vi "ReversedEngineering CreateStateTransationEdges.vi"(1 "GraphRefToAddNodesTo":refnum<class "Graph.lvclass">, 2 "StateDiagramReverseOptions":T1={"Clear All Current States"=TRUE, "UseMenuItem"=TRUE, "InsertArrayQueuedElementsVI"="", "Add Actions"=FALSE, "StateDiagramSerachActions"={"Action"=enum."NotTheseVIs", "VINames"=[], "LimitActions(VIs)"=10}, "AddCaseCommentsAsActions"=FALSE, "IgnoreStatesNotUsed"=FALSE, "CommentsSerachActions"={"MinimumTextLength"=0, "OnlyTopLeftComment"=FALSE, "CommentPrefix"=""}, "TransitionMode"=enum."Add to current transtion text", "ActionMode"=enum."Add to current action text"}, 3 "States":T5[](array[typedef]), 5 "error in (no error)":errorcluster, 7 "graphics":refnum<class "Graphics.lvclass">, 9 "grid":refnum<class "Grid.lvclass">) -> (19 "error out":errorcluster)   [LabVIEW 2014]
uses:
  <resource>/Framework/Providers/Open_GDS/UML/ReversedEngineering/ReversedEngineering StateMachineStateInfo.ctl
  <resource>/Framework/Providers/Open_GDS/UML/Graph_class/Graph.lvclass
  <resource>/Framework/Providers/Open_GDS/UML/Graphics_class/Graphics.lvclass
  <resource>/Framework/Providers/Open_GDS/UML/Grid_class/Grid.lvclass
  <resource>/Framework/Providers/Open_GDS/UML/ReversedEngineering/private/ReversedEngineering StateDiagramReverseOptions.ctl
  <resource>/Framework/Providers/Open_GDS/UML/ReversedEngineering/private/ReversedEngineering StateDiagramSerachActions.ctl
  <resource>/Framework/Providers/Open_GDS/UML/ReversedEngineering/ReversedEngineering StateAnalyseVIAction.ctl
  <resource>/Framework/Providers/Open_GDS/UML/ReversedEngineering/private/ReversedEngineering StateDiagramCommentSearchType.ctl
  <resource>/Framework/Providers/Open_GDS/UML/AbstractEdge_class/AbstractEdge.lvclass
  <resource>/Framework/Providers/Open_GDS/UML/StateNode_class/StateNode.lvclass
  <resource>/Framework/Providers/Open_GDS/UML/StateTransitionEdge_class/StateTransitionEdge.lvclass
  <resource>/Framework/Providers/Open_GDS/UML/MultiLineString_class/MultiLineString.lvclass
  <resource>/Framework/Providers/Open_GDS/UML/AbstractNode_class/AbstractNode.lvclass
  <resource>/Framework/Providers/Open_GDS/UML/StateReverse_class/StateReverse.lvclass
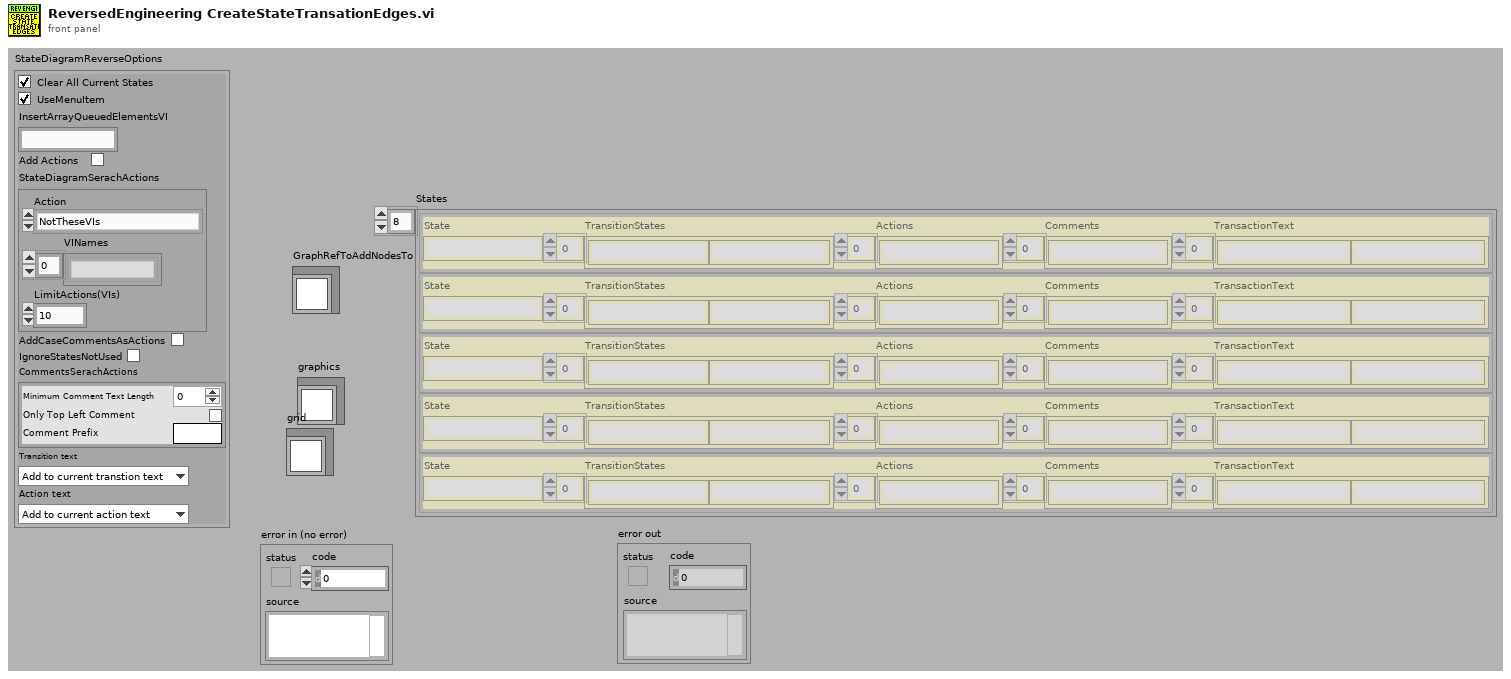
[diagram p1: front panel]
types:
  T1 = typedef "ReversedEngineering StateDiagramReverseOptions.ctl" = cluster{"Clear All Current States":bool, "UseMenuItem":bool, "InsertArrayQueuedElementsVI":string, "Add Actions":bool, "StateDiagramSerachActions":T2, "AddCaseCommentsAsActions":bool, "IgnoreStatesNotUsed":bool, "CommentsSerachActions":T4, "TransitionMode":enum16{"Add to current transtion text", "Replace transition text"}, "ActionMode":enum16{"Add to current action text", "Replace action text"}}
  T2 = typedef "ReversedEngineering StateDiagramSerachActions.ctl" = cluster{"Action":T3, "VINames":string[], "LimitActions(VIs)":i32}
  T3 = typedef "ReversedEngineering StateAnalyseVIAction.ctl" = enum16{"OnlyTheseVIs", "NotTheseVIs"}
  T4 = typedef "ReversedEngineering StateDiagramCommentSearchType.ctl" = cluster{"MinimumTextLength":i32, "OnlyTopLeftComment":bool, "CommentPrefix":string}
  T5 = typedef "ReversedEngineering StateMachineStateInfo.ctl" = cluster{"State":string, "TransitionStates":string[], "Actions":string[], "Comments":string[], "TransactionText":string[]}
  T6 = enum16{"Add to current transtion text", "Replace transition text"}
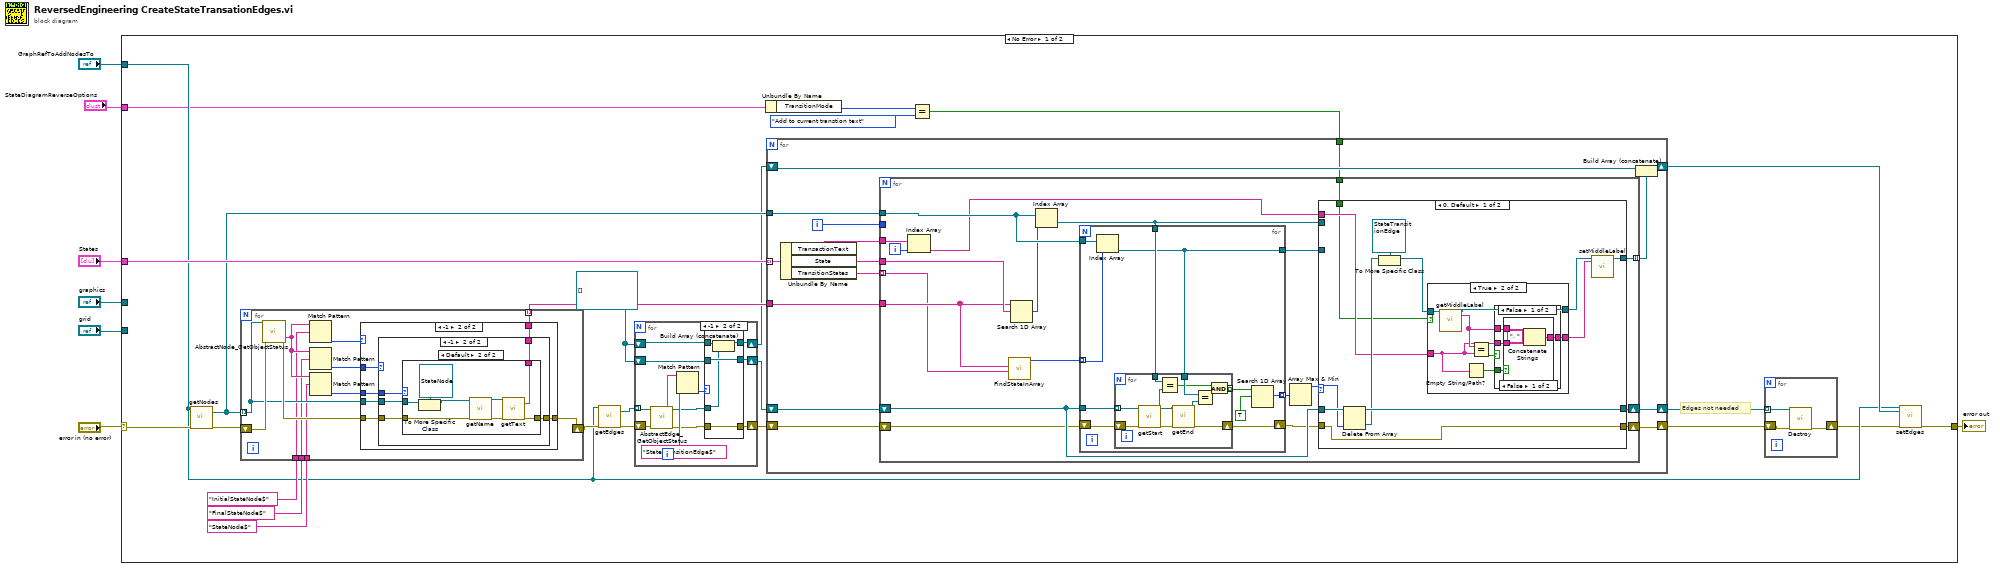
[diagram p0: block diagram]
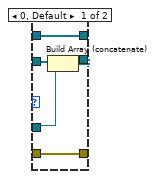
[diagram p2: hidden frame]
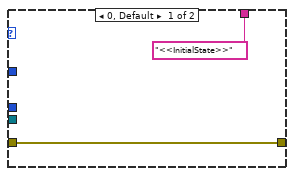
[diagram p3: hidden frame]
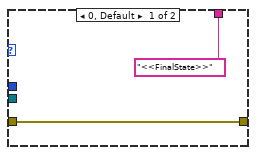
[diagram p4: hidden frame]
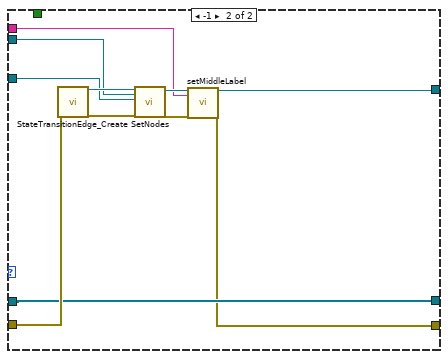
[diagram p9: hidden frame]
diagram:
  n1 = case shown="No Error" "error in (no error)" {
    selector: "error in (no error)" -> [w32 w193]
    tunnel: [w31 w193] -> w6
    tunnel: "States" -> [w30 _]
    tunnel: "GraphRefToAddNodesTo" -> [w21 _]
    tunnel: "graphics" -> [_ _]
    tunnel: "grid" -> [_ _]
    tunnel: "StateDiagramReverseOptions" -> [w11 _]
    frame No Error {
      w13 = refnum<class "AbstractEdge.lvclass">[] []
      # "Edges not needed"
      n2 = call-dynamic "getNodes.vi"("reference"=w21, "error in (no error)"=w32) -> ("nodes"=w29:refnum<class "AbstractNode.lvclass">[], "error out"=w24:errorcluster)  [unwired: 15 in, 1 out]
      n3 = for {
        shift-right: [w66] -> w22
        shift-left: w24 -> [w67]
        tunnel: w29 -> [w64] mode=indexing
        tunnel: [w65] -> w28 mode=indexing
        tunnel: "StateNode$" -> [w63]
        tunnel: "FinalStateNode$" -> [w61]
        tunnel: "InitialStateNode$" -> [w60]
        n4 = call <resource>:"AbstractNode_GetObjectStatus.vi"("reference in"=w64, "error in (no error)"=w67) -> ("Class name"=w62:string, "error out"=w69:errorcluster)  [unwired: 16 out]
        n5 = Match Pattern(string=w62, regular expression=w60) -> (offset past match=w59:i32)  [unwired: 4 out]
        n6 = Match Pattern(string=w62, regular expression=w61) -> (offset past match=w58:i32)  [unwired: 4 out]
        n7 = Match Pattern(string=w62, regular expression=w63) -> (offset past match=w68:i32)  [unwired: 4 out]
        n8 = case shown="-1" w59 {
          tunnel: w69 -> [w70 w77]
          tunnel: w68 -> [_ w76]
          tunnel: [w70 w75] -> w66
          tunnel: ["<<InitialState>>" ("text") w74] -> w65
          tunnel: w64 -> [_ w73]
          tunnel: w58 -> [_ w72]
          frame 0, Default {
          }
          frame -1 {
            n9 = case shown="-1" w72 {
              tunnel: w77 -> [w78 w84]
              tunnel: w76 -> [_ w83]
              tunnel: [w78 w82] -> w75
              tunnel: ["<<FinalState>>" ("text") w81] -> w74
              tunnel: w73 -> [_ w80]
              frame 0, Default {
              }
              frame -1 {
                n10 = case shown="Default" w83 {
                  tunnel: w80 -> [_ w88]
                  tunnel: w84 -> [w85 w93]
                  tunnel: [w85 w90] -> w82
                  tunnel: [_ w89] -> w81
                  frame -1 {
                  }
                  frame Default {
                    n11 = To More Specific Class(target class=refnum<class "StateNode.lvclass"> refnum ("reference"), reference=w88) -> (specific class reference=w86:refnum<class "StateNode.lvclass">)  [unwired: 1 in, 1 out]
                    n12 = call-dynamic "getName.vi"("reference"=w86, "error in (no error)"=w93) -> ("name"=w92:refnum<class "MultiLineString.lvclass">, "error out"=w91:errorcluster)  [unwired: 15 in, 1 out]
                    n13 = call-dynamic "getText.vi"("reference"=w92, "error in (no error)"=w91) -> ("text"=w89:string, "error out"=w90:errorcluster)  [unwired: 15 in, 1 out]
                  }
                }
              }
            }
          }
        }
      }
      n14 = call-dynamic "getEdges.vi"("reference"=w21, "error in (no error)"=w22) -> ("edges"=w16:refnum<class "AbstractEdge.lvclass">[], "error out"=w17:errorcluster)  [unwired: 15 in, 1 out]
      n15 = for {
        tunnel: w16 -> [w44] mode=indexing
        shift-right: [w39] -> w14
        shift-left: w17 -> [w43]
        shift-right: [w35] -> w15
        shift-left: w13 -> [w36]
        shift-right: [w33] -> w12
        shift-left: w13 -> [w34]
        n16 = call <resource>:"AbstractEdge_GetObjectStatus.vi"("reference in"=w44, "error in (no error)"=w43) -> ("Class name"=w42:string, "reference out"=w38:refnum<class "AbstractEdge.lvclass">, "error out"=w40:errorcluster)  [unwired: 15 out]
        n17 = Match Pattern(string=w42, regular expression="StateTransitionEdge$") -> (offset past match=w37:i32)  [unwired: 4 out]
        n18 = case shown="-1" w37 {
          tunnel: w40 -> [w49 w53]
          tunnel: [w49 w53] -> w39
          tunnel: w38 -> [w46 w50]
          tunnel: w36 -> [w48 w54]
          tunnel: [w47 w54] -> w35
          tunnel: w34 -> [w45 w52]
          tunnel: [w45 w51] -> w33
          frame 0, Default {
            n19 = Build Array (concatenate)(w48, w46) -> (w47:refnum<class "AbstractEdge.lvclass">[])
          }
          frame -1 {
            n20 = Build Array (concatenate)(w52, w50) -> (w51:refnum<class "AbstractEdge.lvclass">[])
          }
        }
      }
      n21 = Unbundle By Name(w11) -> ("TransitionMode"=w10:T6)
      n22 = Equal?(x=w10, y=T6."Add to current transtion text") -> (x = y?=w8:bool)
      n23 = for {
        shift-right: [w105] -> w20
        shift-left: w14 -> [w106]
        tunnel: w30 -> [w108] mode=indexing
        tunnel: w29 -> [w104]
        shift-right: [w102] -> w23
        shift-left: w12 -> [w100]
        tunnel: w28 -> [w98]
        shift-right: [w96] -> w19
        shift-left: w15 -> [w97]
        tunnel: w8 -> [w94]
        i -> [w99]
        n24 = Unbundle By Name(w108) -> ("TransactionText"=w95:string[], "State"=w107:string, "TransitionStates"=w103:string[])
        n25 = for {
          tunnel: w107 -> [w125]
          shift-right: [w128] -> w105
          shift-left: w106 -> [w117]
          tunnel: w104 -> [w127]
          tunnel: w103 -> [w114] mode=indexing
          tunnel: [w126] -> w101 mode=indexing
          tunnel: w99 -> [_]
          tunnel: w98 -> [w115]
          shift-right: [w121] -> w96
          shift-left: w97 -> [w120]
          tunnel: w95 -> [w112]
          tunnel: w94 -> [w109]
          i -> [w111]
          n26 = Index Array(array=w112, index=w111) -> (element=w110:string)
          n27 = call <resource>:"FindStateInArray.vi"("TransactionState"=w114, "AllCaseStates"=w115) -> ("AllIndexes"=w113:i32[])  [unwired: 7 in, 2 out]
          n28 = Search 1D Array(1D array=w115, element=w125) -> (index of element=w124:i32)  [unwired: 1 out]
          n29 = Index Array(array=w127, index=w124) -> (element=w123:refnum<class "AbstractNode.lvclass">)
          n30 = for {
            tunnel: w127 -> [w138]
            tunnel: w123 -> [w137]
            tunnel: [w136] -> w122
            tunnel: [w133] -> w119 mode=indexing
            tunnel: w120 -> [w132]
            shift-right: [w131] -> w116
            shift-left: w117 -> [w130]
            tunnel: w113 -> [w129] mode=indexing
            n31 = Index Array(array=w138, index=w129) -> (element=w136:refnum<class "AbstractNode.lvclass">)
            n32 = for {
              shift-right: [w140] -> w131
              shift-left: w130 -> [w149]
              tunnel: w132 -> [w148] mode=indexing
              tunnel: w137 -> [w146]
              tunnel: w136 -> [w143]
              tunnel: [w139] -> w135 mode=indexing
              n33 = call-dynamic "getStart.vi"("reference"=w148, "error in (no error)"=w149) -> ("reference out"=w147:refnum<class "AbstractEdge.lvclass">, "startNode"=w145:refnum<class "AbstractNode.lvclass">, "error out"=w150:errorcluster)  [unwired: 14 in, 1 out]
              n34 = Equal?(x=w146, y=w145) -> (x = y?=w142:bool)
              n35 = call-dynamic "getEnd.vi"("reference"=w147, "error in (no error)"=w150) -> ("endNode"=w144:refnum<class "AbstractNode.lvclass">, "error out"=w140:errorcluster)  [unwired: 14 in, 2 out]
              n36 = Equal?(x=w143, y=w144) -> (x = y?=w141:bool)
              n37 = And(x=w142, y=w141) -> (x .and. y?=w139:bool)
            }
            n38 = Search 1D Array(1D array=w135, element=TRUE) -> (index of element=w133:i32)  [unwired: 1 out]
          }
          n39 = Array Max & Min(array=w119) -> (max value=w118:i32)  [unwired: 3 out]
          n40 = case shown="0, Default" w118 {
            selector: w118 -> [w161 _]
            tunnel: [w159 w183] -> w128
            tunnel: [w156 w185] -> w126
            tunnel: w123 -> [_ w190]
            tunnel: w122 -> [_ w189]
            tunnel: w116 -> [w159 w188]
            tunnel: w120 -> [w162 w187]
            tunnel: [w160 w187] -> w121
            tunnel: w110 -> [w153 w182]
            tunnel: w109 -> [w151 _]
            frame 0, Default {
              n41 = Delete From Array(array=w162, index=w161) -> (deleted portion=w157:refnum<class "AbstractEdge.lvclass">, array with subset deleted=w160:refnum<class "AbstractEdge.lvclass">[])  [unwired: 1 in]
              n42 = To More Specific Class(target class=refnum<class "StateTransitionEdge.lvclass"> refnum ("reference"), reference=w157) -> (specific class reference=w155:refnum<class "StateTransitionEdge.lvclass">)  [unwired: 1 in, 1 out]
              n43 = case shown="True" w151 {
                tunnel: w155 -> [w163 w170]
                tunnel: [w163 w169] -> w154
                tunnel: [w164 w171] -> w152
                tunnel: w153 -> [w164 w166]
                frame False {
                }
                frame True {
                  n44 = call-dynamic "getMiddleLabel.vi"("reference"=w170) -> ("reference out"=w169:refnum<class "StateTransitionEdge.lvclass">, "label"=w168:string)  [unwired: 16 in, 1 out]
                  n45 = Empty String/Path?(string/path=w166) -> (empty?=w165:bool)
                  n46 = Equal?(x=w168, y=w166) -> (x = y?=w167:bool)
                  n47 = case shown="False" w167 {
                    tunnel: [w175 w181] -> w171
                    tunnel: w168 -> [w174 _]
                    tunnel: w166 -> [w173 w181]
                    tunnel: w165 -> [w172 _]
                    frame False {
                      n48 = case shown="False" w172 {
                        tunnel: [w178 w180] -> w175
                        tunnel: w174 -> [w177 w180]
                        tunnel: w173 -> [w176 _]
                        frame False {
                          n49 = Concatenate Strings(w177, ", " ("string"), w176) -> (w178:string)
                        }
                        frame True {
                        }
                      }
                    }
                    frame True {
                    }
                  }
                }
              }
              n50 = call-dynamic "setMiddleLabel.vi"("reference"=w154, "middleLabel"=w152) -> ("reference out"=w156:refnum<class "StateTransitionEdge.lvclass">)  [unwired: 16 in, 1 out]
            }
            frame -1 {
              n51 = call <resource>:"StateTransitionEdge_Create.vi"("error in (no error)"=w188) -> ("reference out"=w192:refnum<class "StateTransitionEdge.lvclass">, "error out"=w191:errorcluster)  [unwired: 1 in, 16 out]
              n52 = call-dynamic "SetNodes.vi"("reference"=w192, "Start"=w190, "End"=w189, "error in (no error)"=w191) -> ("reference out"=w186:refnum<class "StateTransitionEdge.lvclass">, "error out"=w184:errorcluster)  [unwired: 14 in]
              n53 = call-dynamic "setMiddleLabel.vi"("reference"=w186, "middleLabel"=w182, "error in (no error)"=w184) -> ("reference out"=w185:refnum<class "StateTransitionEdge.lvclass">, "error out"=w183:errorcluster)  [unwired: 15 in]
            }
          }
        }
        n54 = Build Array (concatenate)(w100, w101) -> (w102:refnum<class "AbstractEdge.lvclass">[])
      }
      n55 = for {
        shift-right: [w55] -> w18
        shift-left: w20 -> [w57]
        tunnel: w19 -> [w56] mode=indexing
        n56 = call-dynamic "Destroy.vi"("reference"=w56, "error in (no error)"=w57) -> ("error out"=w55:errorcluster)  [unwired: 16 in, 1 out]
      }
      n57 = call-dynamic "setEdges.vi"("reference"=w21, "edges"=w23, "error in (no error)"=w18) -> ("error out"=w31:errorcluster)  [unwired: 15 in, 1 out]
    }
    frame Error {
    }
  }
  "error out" <- w6
